vi "插值.vi"(8 "插值率":dbl, 11 "数字或点的数组":dbl[][](array[numeric])) -> (0 "y值":dbl, 3 "数字或点的数组输出":dbl[][](array[numeric]))   [LabVIEW 2015]
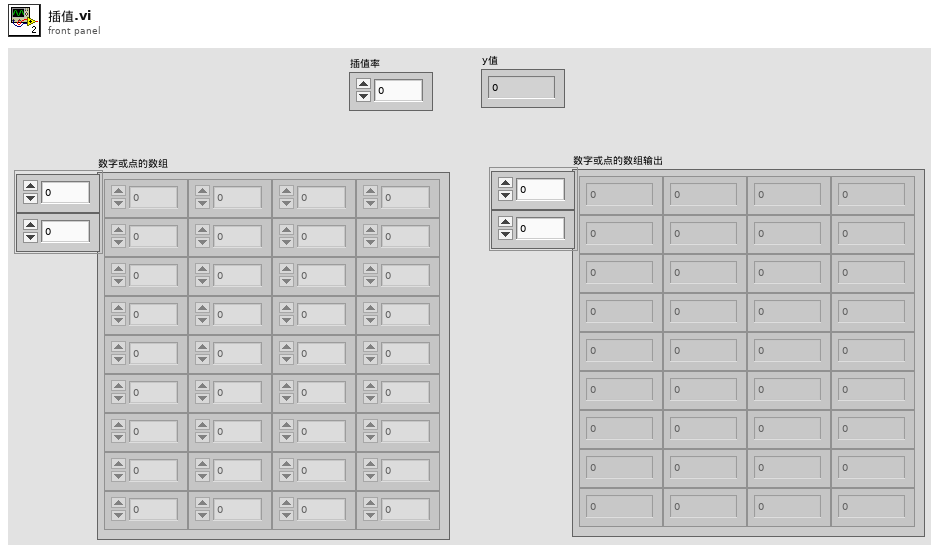
[diagram p1: front panel]
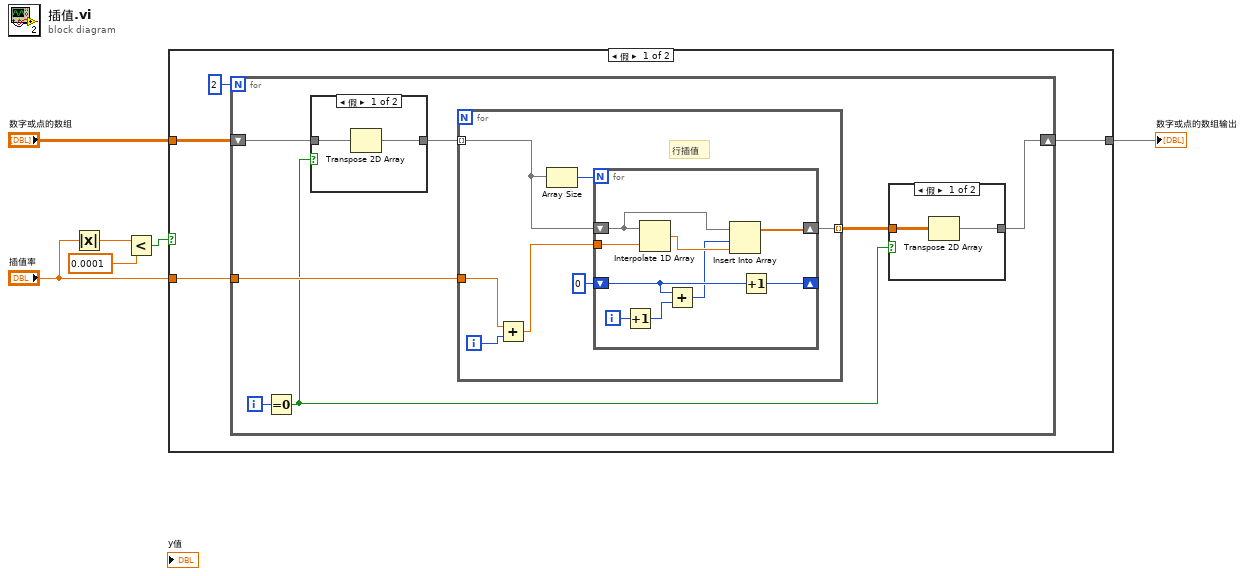
[diagram p0: block diagram]
diagram:
  n1 = Absolute Value(x="插值率") -> (abs(x)=w3:dbl)
  n2 = Less?(x=w3, y=0.0001) -> (x < y?=w1:bool)
  n3 = case shown="假" w1 {
    tunnel: "数字或点的数组" -> [w10 w40]
    tunnel: [w8 w40] -> w5
    tunnel: "插值率" -> [w9 _]
    frame False {
      n4 = for {
        N: 2 -> [_]
        tunnel: w9 -> [w17]
        shift-right: [w11] -> w8
        shift-left: w10 -> [w16]
        i -> [w15]
        n5 = Equal To 0?(x=w15) -> (x = 0?=w13:bool)
        n6 = case shown="假" w13 {
          tunnel: w16 -> [w22 w23]
          tunnel: [w21 w23] -> w14
          frame False {
            n7 = Transpose 2D Array(2D array=w22) -> (transposed array=w21:dbl[][])
          }
          frame True {
          }
        }
        n8 = for {
          tunnel: w14 -> [w27] mode=indexing
          tunnel: [w26] -> w12 mode=indexing
          tunnel: w17 -> [w25]
          i -> [w30]
          # "行插值"
          n9 = Add(x=w25, y=w30) -> (x+y=w29:dbl)
          n10 = Array Size(array=w27) -> (size(s)=w28:i32)
          n11 = for {
            N: w28 -> [_]
            tunnel: w29 -> [w39]
            shift-right: [w35] -> w26
            shift-left: w27 -> [w38]
            shift-right: [w34] -> _
            shift-left: 0 -> [w32]
            i -> [w37]
            n12 = Increment(x=w37) -> (x+1=w33:i32)
            n13 = Interpolate 1D Array(1:w39, 2:w38) -> (0:w36:dbl)
            n14 = Add(x=w32, y=w33) -> (x+y=w31:i32)
            n15 = Insert Into Array(array=w38, index=w31, new element=w36) -> (w35:dbl[])
            n16 = Increment(x=w32) -> (x+1=w34:i32)
          }
        }
        n17 = case shown="假" w13 {
          tunnel: w12 -> [w19 w20]
          tunnel: [w18 w20] -> w11
          frame False {
            n18 = Transpose 2D Array(2D array=w19) -> (transposed array=w18:dbl[][])
          }
          frame True {
          }
        }
      }
    }
    frame True {
    }
  }
  "数字或点的数组输出" <- w5
